vi "DSF.Engine.Framework.Allocate Intermediate Buffer.vi"(8 "error in (no error)":errorcluster, 10 "unallocated Intermediate Buffer":refnum<class "DSF.Engine.Pointer.DBL.lvclass">, 11 "Framework in":refnum<class "DSF.Engine.Framework.lvclass">) -> (0 "error out":errorcluster, 2 "allocated Intermediate Buffer":refnum<class "DSF.Engine.Pointer.DBL.lvclass">, 3 "Framework out":refnum<class "DSF.Engine.Framework.lvclass">)   [LabVIEW 2017, in "DSF.Engine.lvlib" / "DSF.Engine.Framework.lvclass"]
uses:
  DSF.Engine.Framework.lvclass
  Pointer/DSF.Engine.Pointer.DBL.lvclass
  C:/Program Files (x86)/National Instruments/LabVIEW 2017/vi.lib/National Instruments/Memory Manager/Classes/Pointer/Memory.Pointer.lvclass
  <vilib>/National Instruments/Memory Manager/Classes/Pointer/Memory.Pointer.lvclass/Memory.Pointer.ctl
  <vilib>/National Instruments/Memory Manager/Classes/Pointer/Memory.Pointer.lvclass
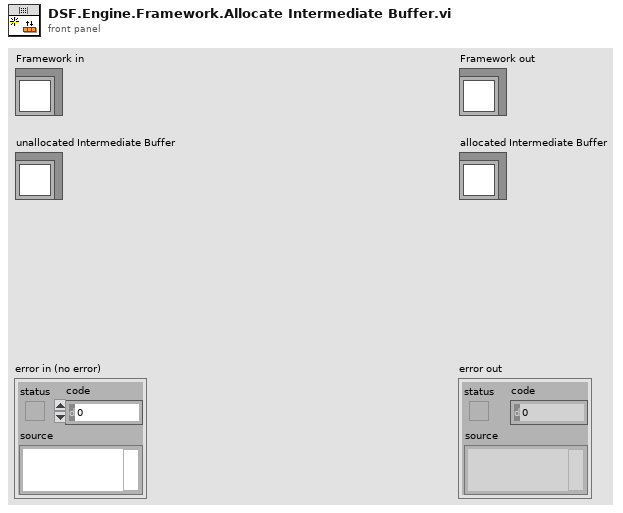
[diagram p1: front panel]
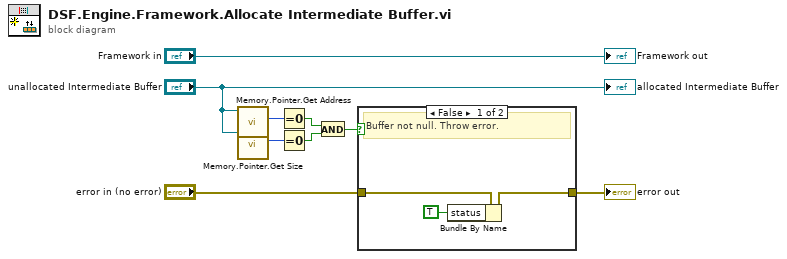
[diagram p0: block diagram]
diagram:
  n1 = call <vilib>:"Memory.Pointer.Get Address.vi"("Pointer in"="unallocated Intermediate Buffer") -> ("address"=w9:u64)  [unwired: 9 in, 1 out]
  n2 = call <vilib>:"Memory.Pointer.Get Size.vi"("Pointer in"="unallocated Intermediate Buffer") -> ("size"=w8:u64)  [unwired: 9 in, 1 out]
  n3 = Equal To 0?(x=w9) -> (x = 0?=w6:bool)
  n4 = Equal To 0?(x=w8) -> (x = 0?=w5:bool)
  n5 = And(x=w6, y=w5) -> (x .and. y?=w3:bool)
  n6 = case shown="False" w3 {
    tunnel: "error in (no error)" -> [w12 w13]
    tunnel: [w11 w13] -> w1
    frame False {
      # "Buffer not null. Throw error."
      n7 = Bundle By Name(cluster=w12, "status"=TRUE) -> (w11:errorcluster)
    }
    frame True {
      # "Buffer is null. Proceed."
    }
  }
  "error out" <- w1
  "Framework out" <- "Framework in"
  "allocated Intermediate Buffer" <- "unallocated Intermediate Buffer"
